vi "Dhoot Top Coordinate System.vi"(0 "Image Out":T7(plugin-control), 1 "Edge Options ROI 1":T4={"Edge Polarity"=0, "Kernel Size"=3, "Width"=3, "Minimum Edge Strength"=10.0, "Interpolation Type"=enum."Bilinear Fixed", "Data Processing Method"=enum."Average"} {"Edge Polarity" items=["All Edges", "Rising Edges", "Falling Edges"]; "Minimum Edge Strength" format="%.2f"; "Width" step=2; "Kernel Size" step=2}, 2 "Edge Options ROI 2":T4={"Edge Polarity"=0, "Kernel Size"=3, "Width"=3, "Minimum Edge Strength"=10.0, "Interpolation Type"=enum."Bilinear Fixed", "Data Processing Method"=enum."Average"} {"Edge Polarity" items=["All Edges", "Rising Edges", "Falling Edges"]; "Minimum Edge Strength" format="%.2f"; "Width" step=2; "Kernel Size" step=2}, 3 "Line Options ROI 1":T2={"Number of Lines"=1, "Type"=enum."First Edge Rake", "Min. Score"=10.0, "Max. Score"=1000.0, "Orientation"=0.0, "Angle Range"=45.0, "Angle Tolerance"=1.0, "Step Size"=7, "Min. SNR (db)"=0.0, "Min. Points (%)"=25.0, "Hough Iterations"=5} {"Min. Points (%)" min=0.0 max=100.0; "Min. SNR (db)" min=0.0; "Max. Score" min=0.0 max=1024.0; "Min. Score" min=0.0 max=1024.0 step=1.0}, 4 "Line Options ROI 2":T2={"Number of Lines"=1, "Type"=enum."First Edge Rake", "Min. Score"=10.0, "Max. Score"=1000.0, "Orientation"=0.0, "Angle Range"=45.0, "Angle Tolerance"=1.0, "Step Size"=7, "Min. SNR (db)"=0.0, "Min. Points (%)"=25.0, "Hough Iterations"=5} {"Min. Points (%)" min=0.0 max=100.0; "Min. SNR (db)" min=0.0; "Max. Score" min=0.0 max=1024.0; "Min. Score" min=0.0 max=1024.0 step=1.0}, 5 "error in (no error)":errorcluster, 6 "ROI 1":T1 {"Contours"."Type" items=["No Selection", "Point", "Line", "Rectangle", "Oval", "Polygon", "Free", "Annulus", "Unused2", "Unused3", "Broken Line", "Free Hand Line", "Rotated Rectangle"]}, 7 "Search Direction ROI 1":u32, 8 "ROI 2":T1 {"Contours"."Type" items=["No Selection", "Point", "Line", "Rectangle", "Oval", "Polygon", "Free", "Annulus", "Unused2", "Unused3", "Broken Line", "Free Hand Line", "Rotated Rectangle"]}, 9 "Search Direction ROI 2":u32) -> (14 "Co ordinate System":T6, 19 "error out":errorcluster)   [LabVIEW 2019, in "Algorithm.lvclass"]
uses:
  FrameworkOverrides/Algorithm.lvclass
  <vilib>/vision/NI_Vision_Development_Module.lvlib
  <vilib>/vision/Measure.llb/Edge Polarity.ctl
  <vilib>/vision/Measure.llb/Edge Options.ctl
  <vilib>/vision/Measure.llb/Straight Edge Process.ctl
  <vilib>/vision/Measure.llb/Straight Edge Options.ctl
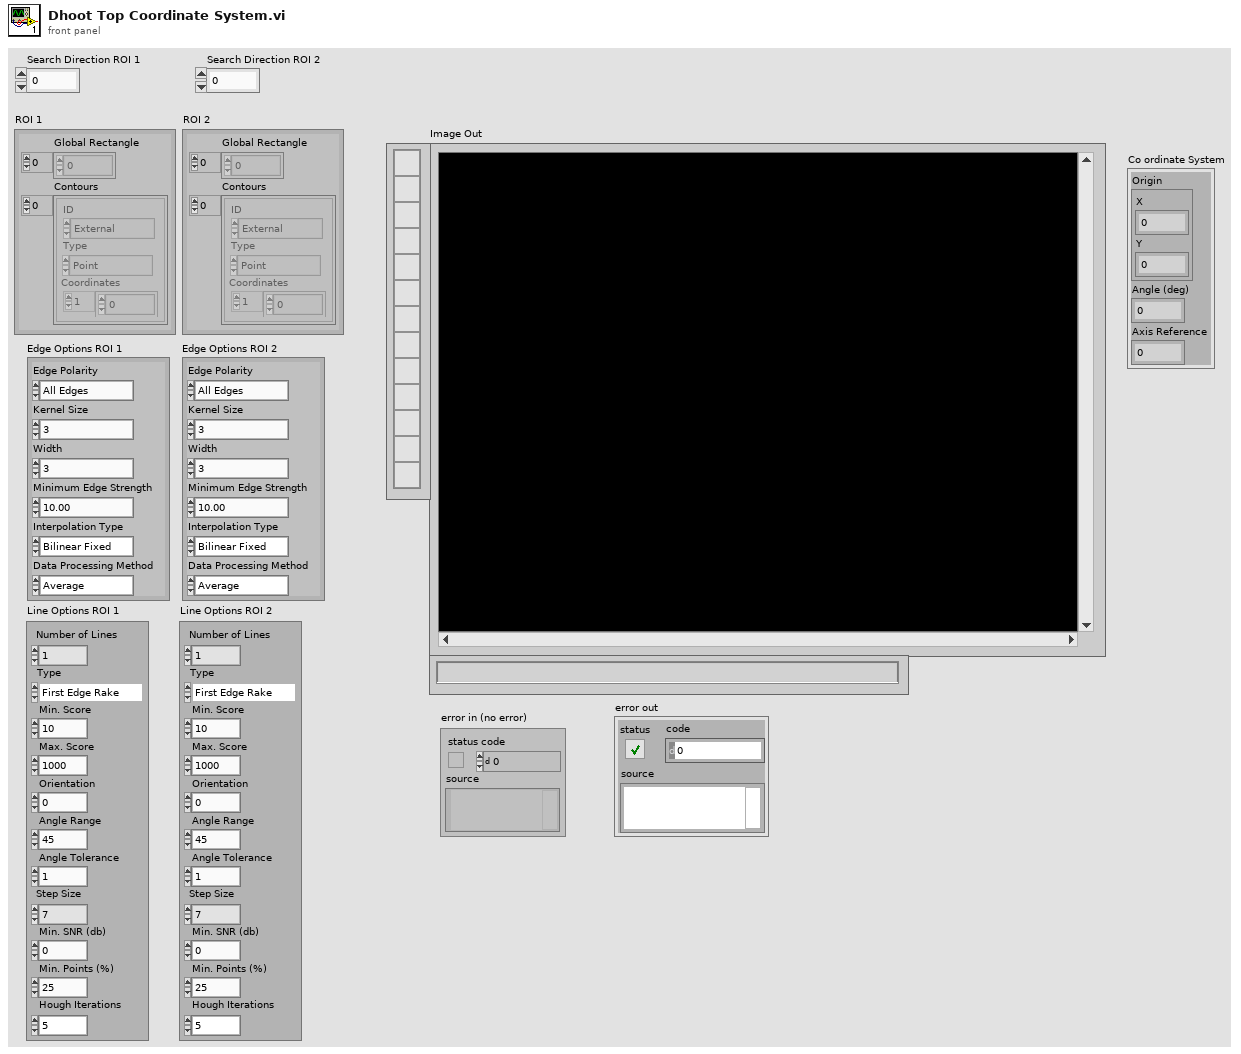
[diagram p1: front panel]
types:
  T1 = cluster{"Global Rectangle":i32[], "Contours":cluster{"ID":enum32{"External", "Internal"}, "Type":u32, "Coordinates":i32[]}[]}
  T2 = typedef "Straight Edge Options.ctl" = cluster{"Number of Lines":i32, "Type":T3, "Min. Score":dbl, "Max. Score":dbl, "Orientation":dbl, "Angle Range":dbl, "Angle Tolerance":dbl, "Step Size":u32, "Min. SNR (db)":dbl, "Min. Points (%)":dbl, "Hough Iterations":i32}
  T3 = typedef "Straight Edge Process.ctl" = enum32{"First Edge Rake", "Best Edge Rake", "Hough Edge Rake", "First Edge Projection", "Best Edge Projection"}
  T4 = typedef "Edge Options.ctl" = cluster{"Edge Polarity":T5, "Kernel Size":u32, "Width":u32, "Minimum Edge Strength":sgl, "Interpolation Type":enum32{"Zero Order", "Bilinear", "Quadratic", "Cubic", "Bilinear Fixed"}, "Data Processing Method":enum32{"Average", "Median"}}
  T5 = typedef "Edge Polarity.ctl" = u32
  T6 = cluster{"Origin":cluster{"X":sgl, "Y":sgl}, "Angle (deg)":sgl, "Axis Reference":u32}
  T7 = typedef "IMAQ Image.ctl" = refnum<image>
  T8 = cluster{"Search Direction":u32, "Edge Options":T4, "Show Search Area":bool, "Show Search Lines":bool, "Show Edges Found":bool, "Show Result":bool, "Search Area Color":u32, "Search Lines Color":u32, "Edge Locations Color":u32, "Result Color":u32, "Overlay Group Name":string}
  T9 = cluster{"Point1 (Pixels)":cluster{"X":sgl, "Y":sgl}, "Point2 (Pixels)":cluster{"X":sgl, "Y":sgl}, "Point1 (Real-World)":cluster{"X":sgl, "Y":sgl}, "Point2 (Real-World)":cluster{"X":sgl, "Y":sgl}, "Angle (Pixel)":dbl, "Angle (Real-World)":dbl, "Score":dbl, "Straightness":dbl, "Average SNR (db)":dbl, "Calibration Valid":bool}[]
  T10 = cluster{"Point1 (Pixels)":cluster{"X":sgl, "Y":sgl}, "Point2 (Pixels)":cluster{"X":sgl, "Y":sgl}, "Point1 (Real-World)":cluster{"X":sgl, "Y":sgl}, "Point2 (Real-World)":cluster{"X":sgl, "Y":sgl}, "Angle (Pixel)":dbl, "Angle (Real-World)":dbl, "Score":dbl, "Straightness":dbl, "Average SNR (db)":dbl, "Calibration Valid":bool}
  T11 = cluster{"Point1 (Pixels)":cluster{"X":sgl, "Y":sgl}, "Point2 (Pixels)":cluster{"X":sgl, "Y":sgl}}
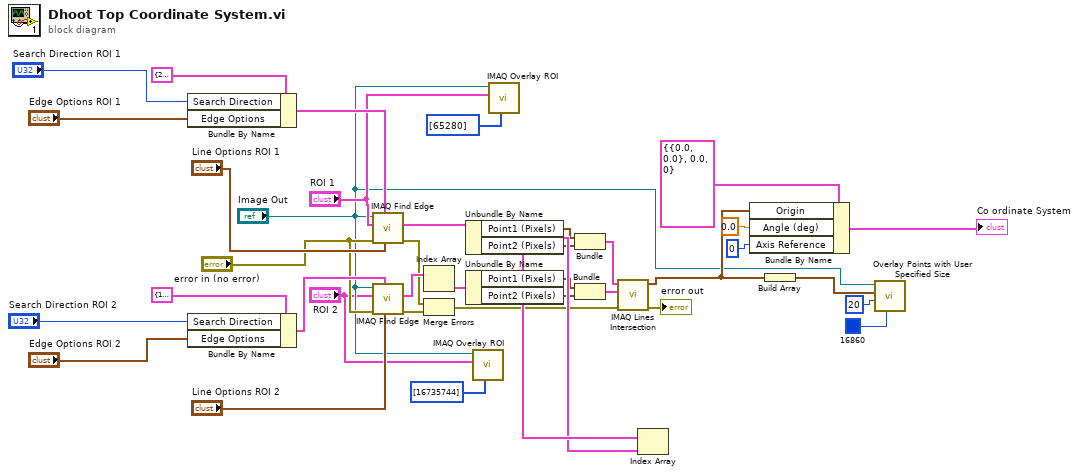
[diagram p0: block diagram]
diagram:
  n1 = Bundle By Name(cluster=T8 {"Search Direction"=2, "Edge Options"={"Edge Polarity"=0, "Kernel Size"=5, "Width"=5, "Minimum Edge Strength"=50.0, "Interpolation Type"=enum."Bilinear Fixed", "Data Processing Method"=enum."Average"}, "Show Search Area"=FALSE, "Show Search Lines"=FALSE, "Show Edges Found"=FALSE, "Show Result"=TRUE, "Search Area Color"=65280, "Search Lines Color"=255, "Edge Locations Color"=16776960, "Result Color"=16711680, "Overlay Group Name"=""} ("Options"), "Search Direction"="Search Direction ROI 1", "Edge Options"="Edge Options ROI 1") -> (w12:T8)
  n2 = Bundle By Name(cluster=T8 {"Search Direction"=1, "Edge Options"={"Edge Polarity"=0, "Kernel Size"=5, "Width"=5, "Minimum Edge Strength"=50.0, "Interpolation Type"=enum."Zero Order", "Data Processing Method"=enum."Average"}, "Show Search Area"=FALSE, "Show Search Lines"=FALSE, "Show Edges Found"=FALSE, "Show Result"=TRUE, "Search Area Color"=65280, "Search Lines Color"=255, "Edge Locations Color"=16776960, "Result Color"=16711680, "Overlay Group Name"=""} ("Options"), "Search Direction"="Search Direction ROI 2", "Edge Options"="Edge Options ROI 2") -> (w8:T8)
  n3 = call "IMAQ Find Edge"("Line Fit Options"="Line Options ROI 1", "Options"=w12, "error in (no error)"="error in (no error)", "ROI Descriptor"="ROI 1", "Image"="Image Out") -> ("error out"=w26:errorcluster, "Straight Edges"=w36:T9)  [unwired: 3 in, 2 out]
  n4 = call "IMAQ Find Edge"("Line Fit Options"="Line Options ROI 2", "Options"=w8, "error in (no error)"="error in (no error)", "ROI Descriptor"="ROI 2", "Image"="Image Out") -> ("error out"=w25:errorcluster, "Straight Edges"=w35:T9)  [unwired: 3 in, 2 out]
  n5 = Index Array(array=w35) -> (element=w33:T10)  [unwired: 1 in]
  n6 = Merge Errors(w26, w25) -> (w24:errorcluster)
  n7 = Unbundle By Name(w33) -> ("Point1 (Pixels)"=w29:cluster{"X":sgl, "Y":sgl}, "Point2 (Pixels)"=w28:cluster{"X":sgl, "Y":sgl})
  n8 = call "IMAQ Overlay ROI"("Colors (Green)"=u32[] [16735744], "ROI Descriptor"="ROI 2", "Image"="Image Out") -> ()  [unwired: 7 in, 2 out]
  n9 = call "IMAQ Overlay ROI"("Colors (Green)"=u32[] [65280], "ROI Descriptor"="ROI 1", "Image"="Image Out") -> ()  [unwired: 7 in, 2 out]
  n10 = Bundle("Point1 (Pixels)"=w29, "Point2 (Pixels)"=w28) -> (w27:T11)  [unwired: 1 in]
  n11 = Index Array(array=w36) -> (element=w34:T10)  [unwired: 1 in]
  n12 = Unbundle By Name(w34) -> ("Point1 (Pixels)"=w32:cluster{"X":sgl, "Y":sgl}, "Point2 (Pixels)"=w31:cluster{"X":sgl, "Y":sgl})
  n13 = Bundle("Point1 (Pixels)"=w32, "Point2 (Pixels)"=w31) -> (w30:T11)  [unwired: 1 in]
  n14 = call "IMAQ Lines Intersection"("error in (no error)"=w24, "Line 2"=w27, "Line 1"=w30) -> ("error out"=→"error out":errorcluster, "Intersection Point"=w19:cluster{"X":sgl, "Y":sgl})  [unwired: 6 in, 1 out]
  n15 = Bundle By Name(cluster=T6 {"Origin"={"X"=0.0, "Y"=0.0}, "Angle (deg)"=0.0, "Axis Reference"=0} ("Coordinate System"), "Origin"=w19, "Angle (deg)"=sgl 0.0, "Axis Reference"=u32 0) -> (→"Co ordinate System":T6)
  n16 = Build Array(w19) -> (w18:cluster{"X":sgl, "Y":sgl}[])
  n17 = call "Overlay Points with User Specified Size.vi"("Color"=u32 16860, "Point Diameter (5)"=u32 20, "Points"=w18, "Image In"="Image Out") -> ()  [unwired: 6 in, 2 out]
